vi "002BH_pH_串口地址写入.vi"(8 "error in (no error)":errorcluster caption="错误输入（无错误）", 10 "数值":u16, 11 "MB_Serial session in":refnum<class "MB_Master_Serial.lvclass">) -> (0 "error out":errorcluster caption="错误输出", 3 "MB_Serial session out":refnum<class "MB_Master_Serial.lvclass">)   [LabVIEW 2016, in "国弘多参数.lvlib"]
uses:
  <vilib>/Plasmionique/MB Master/MB_Master_Serial/MB_Master_Serial.lvclass
  C:/Program Files (x86)/National Instruments/LabVIEW 2016/vi.lib/Plasmionique/MB Master/MB_Master/MB_Master.lvclass
  <vilib>/Plasmionique/MB Master/MB Master.lvlib
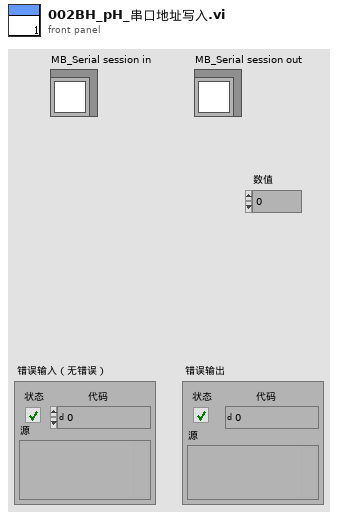
[diagram p1: front panel]
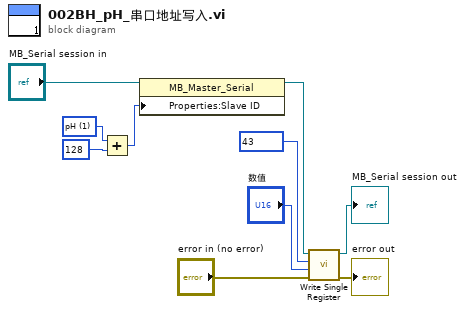
[diagram p0: block diagram]
diagram:
  w5 = u16 1 items=["NULL", "pH", "Cond", "DO", "Turb"] ("数值")
  n1 = Add(x=w5, y=u16 128) -> (x+y=w4:u16)
  n2 = property class="MB_Master_Serial"(reference="MB_Serial session in", "Properties:Slave ID"=w4) -> (reference out=w1:refnum<class "MB_Master_Serial.lvclass">)  [unwired: 1 in, 1 out]
  n3 = call <vilib>:"Write Single Register.vi"("error in (no error)"="error in (no error)", "value"="数值", "address"=u16 43 ("starting address"), "MB session in"=w1) -> ("error out"=→"error out":errorcluster, "MB session out"=→"MB_Serial session out":refnum<class "MB_Master_Serial.lvclass">)  [unwired: 6 in]
